vi "Target B to voltage.vi"(0 "B_x":dbl, 5 "B_y":dbl, 7 "B_z":dbl, 9 "Earth B_x":dbl, 11 "Earth B_y":dbl, 12 "Earth B_z":dbl) -> (4 "element":dbl, 6 "element 2":dbl, 8 "element 3":dbl)   [LabVIEW 2012]
uses:
  <vilib>/Analysis/Matrix/Datatypes/RealMatrix.ctl
  <vilib>/Analysis/baseanly.llb/Real Inverse Matrix.vi
  <vilib>/Analysis/Matrix/Numeric/Subtract/Subtract - RM,RM.vi
  <vilib>/Analysis/baseanly.llb/Real A x B.vi
  <vilib>/Analysis/NI_AALBase.lvlib
  <vilib>/Analysis/Matrix/NI_Matrix.lvlib
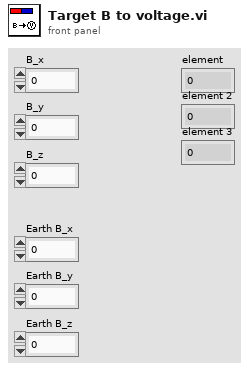
[diagram p1: front panel]
types:
  T1 = typedef "NI_Matrix.lvlib/RealMatrix.ctl" = dbl[][]
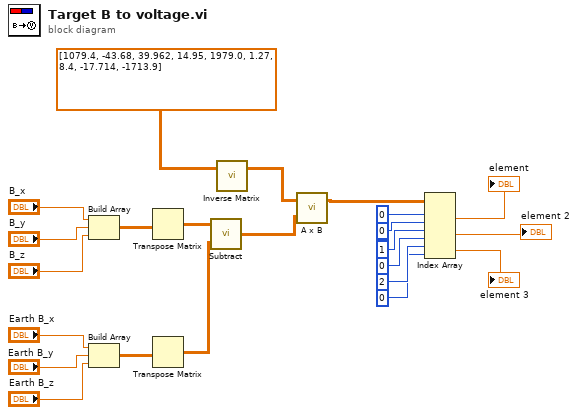
[diagram p0: block diagram]
diagram:
  n1 = Build Array("B_x", "B_y", "B_z") -> (w17:T1)
  n2 = Build Array("Earth B_x", "Earth B_y", "Earth B_z") -> (w12:T1)
  n3 = Transpose Matrix(1:w17) -> (0:w16:T1)
  n4 = Transpose Matrix(1:w12) -> (0:w11:T1)
  n5 = call-poly <vilib>:"Subtract.vi"("Real Matrix B"=w11, "Real Matrix A"=w16) -> ("A - B"=w21:T1)
  n6 = call-poly <vilib>:"Inverse Matrix.vi"("Input Matrix"=T1 [[1079.4, -43.68, 39.962], [14.95, 1979.0, 1.27], [8.4, -17.714, -1713.9]]) -> ("Inverse Matrix"=w22:T1)  [unwired: 1 in, 1 out]
  n7 = call-poly <vilib>:"A x B.vi"("B"=w21, "A"=w22) -> ("A x B"=w10:T1)  [unwired: 1 out]
  n8 = Index Array(array=w10, index (row) #1=0 ("index (row)"), index (col) #1=0 ("index (col)"), index (row) #2=1 ("index (row)"), index (col) #2=0 ("index (col)"), index (row) #3=2 ("index (row)"), index (col) #3=0 ("index (col)")) -> (element #1=→"element":dbl, element #2=→"element 2":dbl, element #3=→"element 3":dbl)
